vi "straight_drive.vi"(8 "Initial Drive Power":dbl, 9 "Right Encoder Speed":dbl, 10 "Left Encoder Speed":dbl) -> (1 "Left Drive PWM":dbl, 2 "Right Drive PWM":dbl)   [LabVIEW 2011]
panel:
  in  "Velocity Gain":dbl
  out "Velocity Error":dbl
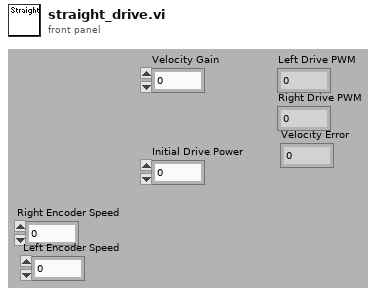
[diagram p1: front panel]
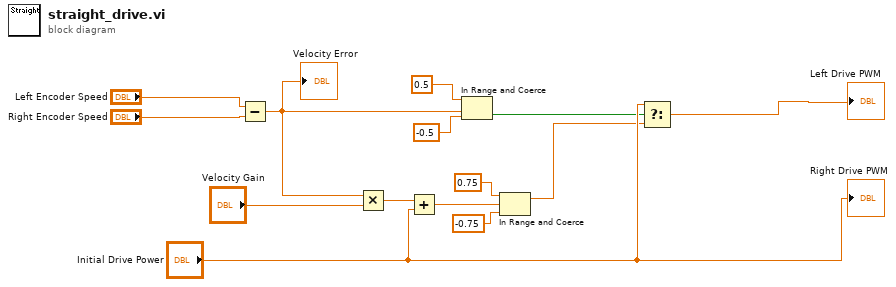
[diagram p0: block diagram]
diagram:
  n1 = Subtract(x="Left Encoder Speed", y="Right Encoder Speed") -> (x-y=w4:dbl)
  "Velocity Error" <- w4
  n2 = Multiply(x=w4, y="Velocity Gain") -> (x*y=w6:dbl)
  n3 = Add(x=w6, y="Initial Drive Power") -> (x+y=w5:dbl)
  n4 = In Range and Coerce(upper limit=0.5, x=w4, lower limit=-0.5) -> (In Range?=w11:bool)  [unwired: 1 out]
  n5 = In Range and Coerce(upper limit=0.75, x=w5, lower limit=-0.75) -> (coerced(x)=w12:dbl)  [unwired: 1 out]
  n6 = Select(t="Initial Drive Power", s=w11, f=w12) -> (s? t:f=→"Left Drive PWM":dbl)
  "Right Drive PWM" <- "Initial Drive Power"
